vi "Spec Add.vi"(7 "프런트패널 윈도우:동작":T1(ring)=enum."Default", 8 "error in":errorcluster caption="에러 입력(에러 없음)", 11 "TBCALSPEC":string[][](table)) -> (0 "error out":errorcluster caption="에러 출력")   [LabVIEW 2020]
uses:
  Controls/Cmd_Spec Add.ctl
  Controls/Cmd_Mouse Popup.ctl
  Controls/Cmd_Read Query.ctl
  Controls/Clst_Query Info.ctl
  Controls/Cmd_Write Query.ctl
  <vilib>/Utility/miscctls.llb/LVRowAndColumnUnsignedTypeDef.ctl
  Variables/Global_Cal Info.vi
  Public/Polymorph/Array Dedup_1D Str.vi
  Public/Polymorph/Cell Space_Table.vi
  Public/Polymorph/Data Class_2D Str.vi
  <vilib>/addons/database/NI_Database_API.lvlib
panel:
  in  "번호정렬":bool
  in  "DB수정":bool
  in  "내용적용":bool
  in  "zero?":bool=TRUE caption="0점 10 digit 추가?"
  out "Data source":string[][](array[string])
  out "추가배열":string[](array[string])
  in  "새로 고침":bool
  in  "등록번호":string
  in  "빈칸\n줄임":bool
  in  "세부교정기능":string(combo)
  in  "교정기능":string(combo)
  in  "추가":bool
  in  "닫기":bool
  out "제조사명":string
  in  "제조사코드":string
  in  "모델":string
  out "기관명":string
  in  "DB등록":bool
  out "세부분류코드":string
  out "부서명":string
  in  "부서코드":string
  in  "기관코드":string
  in  "추가 단위":string(combo)
  in  "추가SPEC":string
  in  "Default 단위":string(combo)
  in  "Default 값":string
  out "슬라이드":i32(slide) scale=0.0..643.0
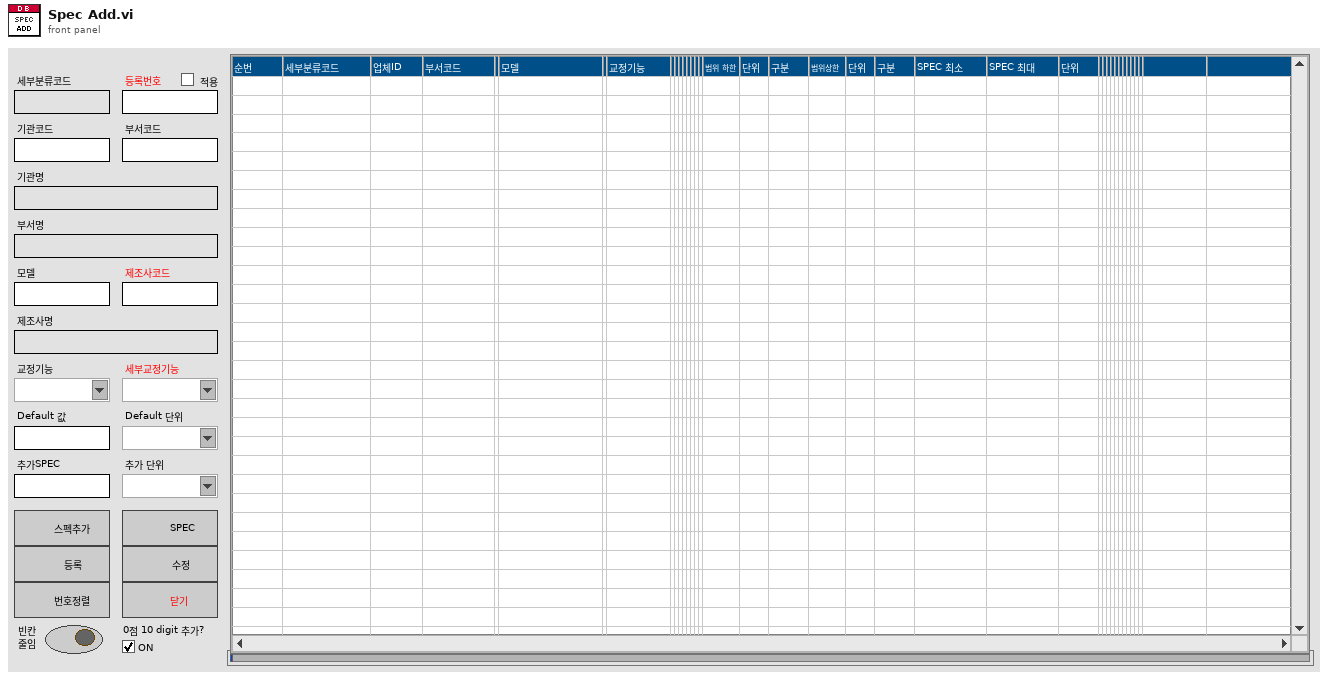
[diagram p1: front panel]
types:
  T1 = enum32{"Invalid", "Default", "Floating", "Floating/Auto-Hide", "Modal"}
  T2 = typedef "Cmd_Spec Add.ctl" = enum16{"Initialize", "Load Spec", "Wait Event", "Check data", "Create Row", "Add Spec", "Update Spec", "Error", "Exit"}
  T3 = typedef "Cmd_Mouse Popup.ctl" = enum16{"활성화", "메뉴선택"}
  T4 = cluster{"Shift":bool, "Ctrl":bool, "Alt":bool, "Cmd":bool, "Opt":bool}
  T5 = typedef "Clst_Query Info.ctl" = cluster{"사번":string, "등록번호":string, "업체명":string, "세부분류코드":string, "형식":string, "기기번호":string, "FUNC":string, "FUNC_EXT":string, "옵션":string, "추가문자열":string, "일자":string, "배열 1":string[], "배열 2":string[], "항목명":string, "문자열":string, "이름":string}
  T6 = typedef "Cmd_Read Query.ctl" = enum16{"교정자 이름 얻기", "인증교정자 얻기", "기술책임자 얻기", "기책부책 얻기", "등록번호 얻기", "등록정보 얻기", "업체정보 얻기", "교정일자(CAMAS) 얻기", "교정일자(CALSTD) 얻기", "교정환경 얻기", "교정절차서 목록 얻기", "교정절차서명 얻기", "교정절차 목록얻기", "교정절차 얻기", "PROC 교정절차 얻기", "PROC SPEC 얻기", "교정절차(Func별) 얻기", "교정절차(Func_ext별) 얻기", "기관코드 얻기", "교정기능(세부분류) 얻기", "교정기능(모델) 얻기", "교정기능 목록 얻기", "교정기능 명칭 얻기", "교정기능 항목명칭 얻기", "DB (사용기준기) 얻기", "DB (기준기이름) 얻기", "DB (기준기이름목록) 얻기", "DB (기준기목록) 얻기", "DB (기준기값) 얻기", "DB (CMC) 얻기", "DB (FUNC) 얻기", "DB (CALNAME) 얻기", "DB (STDNAME) 얻기", "DB (SPEC) 얻기", "모델(항목전체) 얻기", "모델(최대범위) 얻기", "모델(최소범위) 얻기", "모델(최대최소) 얻기", "모델(범위조건) 얻기", "모델(등록요청) 얻기", "모델(형식별) 얻기", "모델(조건별) 얻기", "모델(모델검색) 얻기", "세부분류 목록 얻기", "기준기등록리스트 얻기", "STD Cal Date Check", "DB등록일자 얻기", "적용항목 얻기", "기타정보 얻기", "기준기요청 얻기", "서버버전 얻기"}
  T7 = typedef "Cmd_Write Query.ctl" = enum16{"TBUSESTD_MCT Insert", "TBUSESTD_MCT Delete", "TBCALSTD_MCT_TEMP Insert", "TBCALSTD_MCT_TEMP Delete", "TBCALSTD_MCT Insert", "TBCALSTD_MCT Delete", "TBCALSTD_MCT_BACK Insert", "TBCALSTD_MCT_BACK Delete", "TBCALPROC_MCT Insert", "TBCALPROC_MCT Delete", "TBCALPROC_MCT_TEMP Insert", "TBCALPROC_MCT_TEMP Delete", "TBCALCMC_MCT Insert", "TBCALCMC_MCT Delete", "TBCALFUNC_MCT Insert", "TBCALFUNC_MCT Delete", "TBCALNAME_MCT Insert", "TBCALNAME_MCT Delete", "TBSTDNAME_MCT Insert", "TBSTDNAME_MCT Delete", "TBCALSPEC_MCT Insert", "TBCALSPEC_MCT Delete", "TBCALSTD_MCT NOTUSE update", "TBCALSPEC_MCT update", "TBMCTVERMAN update"}
  T8 = typedef "LVRowAndColumnUnsignedTypeDef.ctl" = cluster{"Row":u32, "Column":u32}
  T9 = typedef "Clst_Cal Info Global.ctl" = cluster{"등록번호":string, "의뢰기관":string, "기기명":string, "제작회사":string, "형식":string, "기기번호":string, "소분류코드":string, "세부분류코드":string, "교정주기":string, "접수번호":string, "교정일자":string, "교정절차서 1":string, "교정절차서 2":string, "교정절차서 3":string, "접수확인자":string, "인증교정자":string, "기술책임자":string, "KOLAS 유무":string, "진행상태":string, "의뢰기관코드":string, "입고형태":string, "영문성적서?":bool, "합불판정?":bool, "부록?":bool, "절차서번호 1":string, "절차서번호 2":string, "절차서번호 3":string, "교정방식":string, "부서명":string}
  T10 = typedef "NI_Database_API.lvlib/Conn ObjectReference.ctl" = refnum<k1>
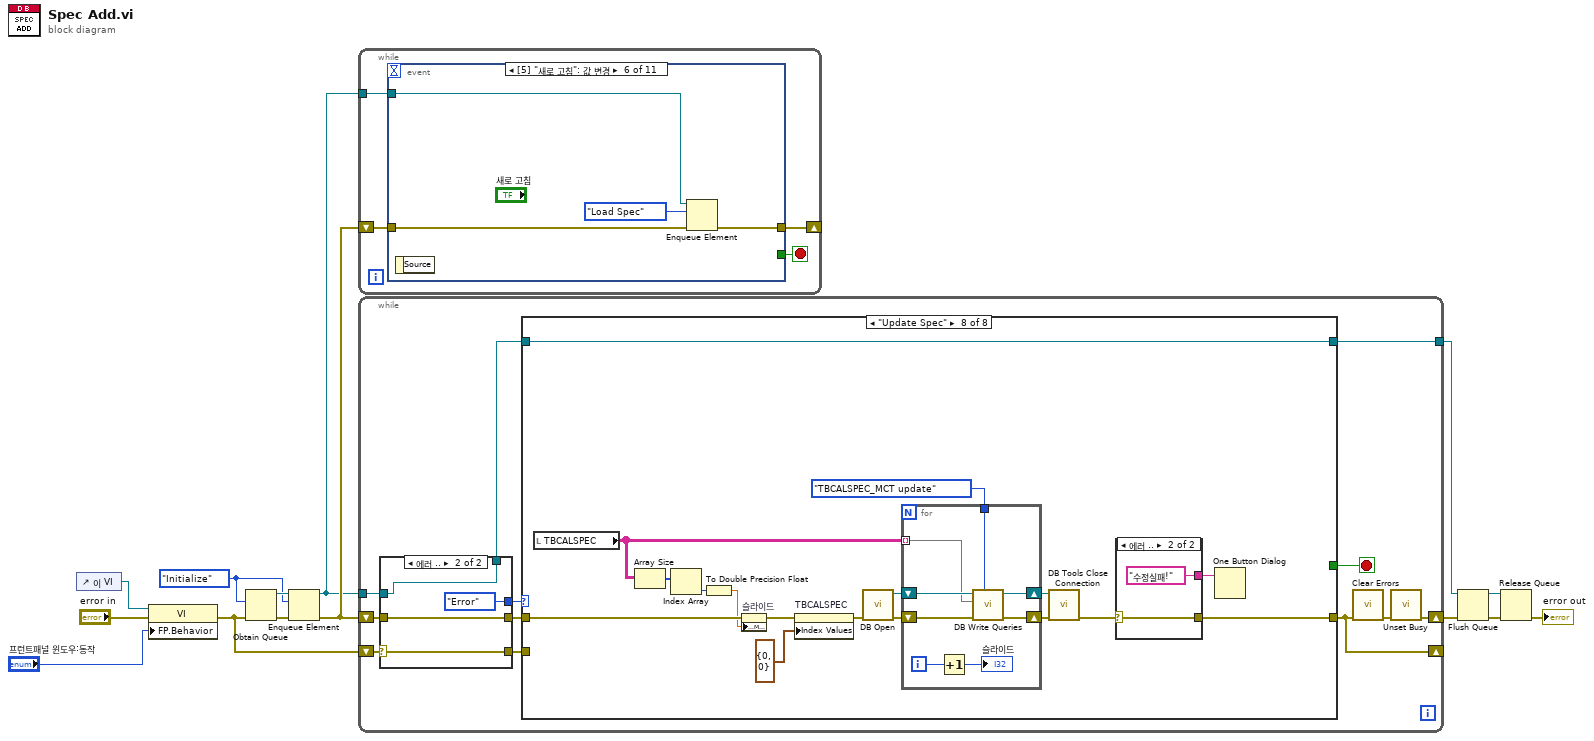
[diagram p0: block diagram]
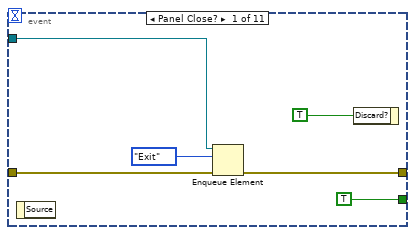
[diagram p2: hidden frame]
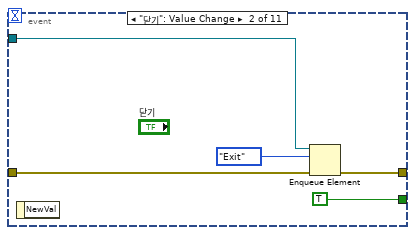
[diagram p3: hidden frame]
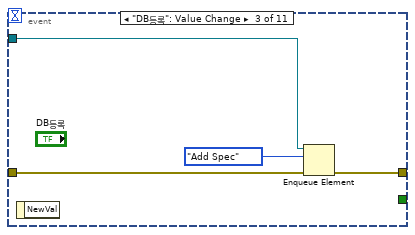
[diagram p4: hidden frame]
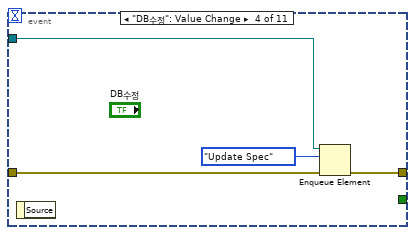
[diagram p5: hidden frame]
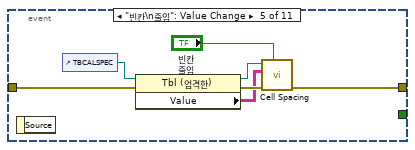
[diagram p6: hidden frame]
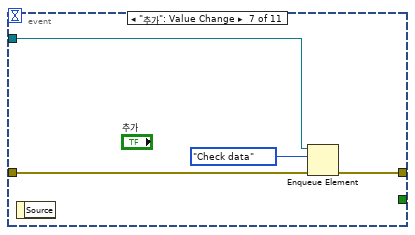
[diagram p7: hidden frame]
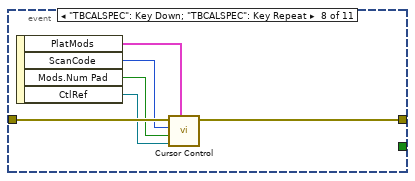
[diagram p8: hidden frame]
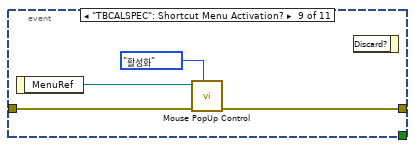
[diagram p9: hidden frame]
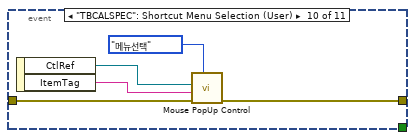
[diagram p10: hidden frame]
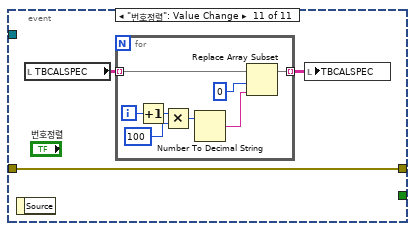
[diagram p11: hidden frame]
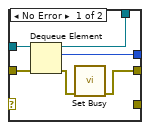
[diagram p12: hidden frame]
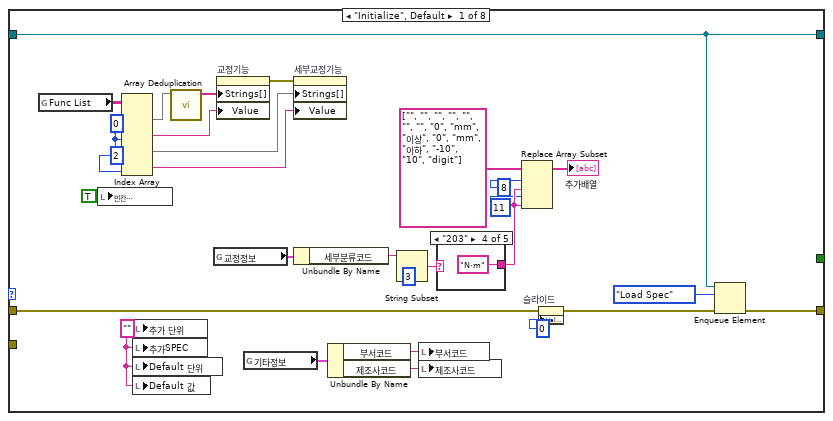
[diagram p13: hidden frame]
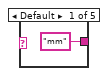
[diagram p14: hidden frame]
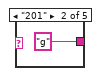
[diagram p15: hidden frame]
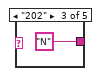
[diagram p16: hidden frame]
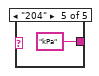
[diagram p17: hidden frame]
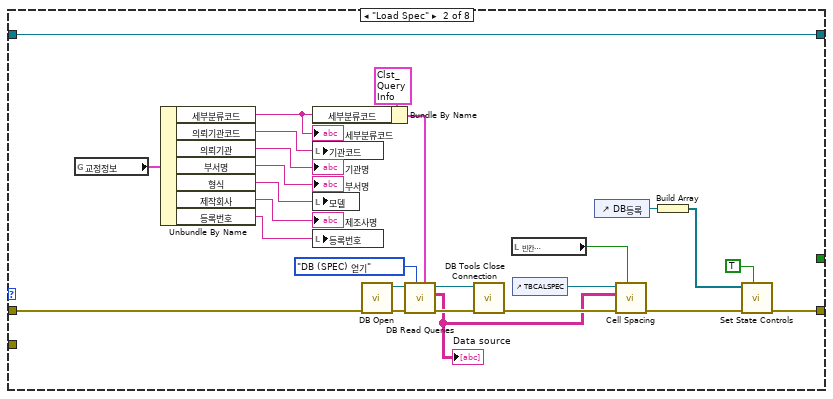
[diagram p18: hidden frame]
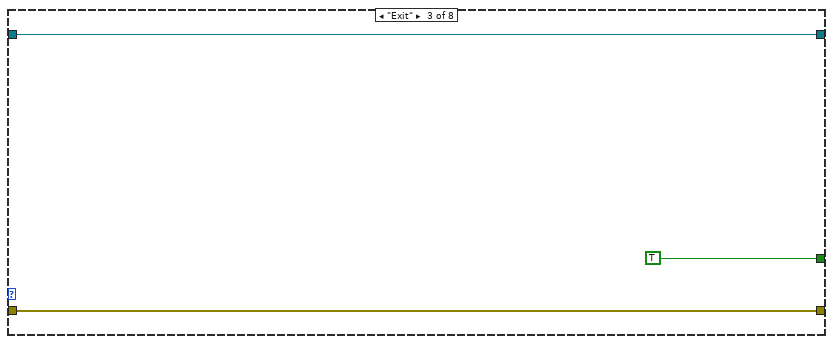
[diagram p19: hidden frame]
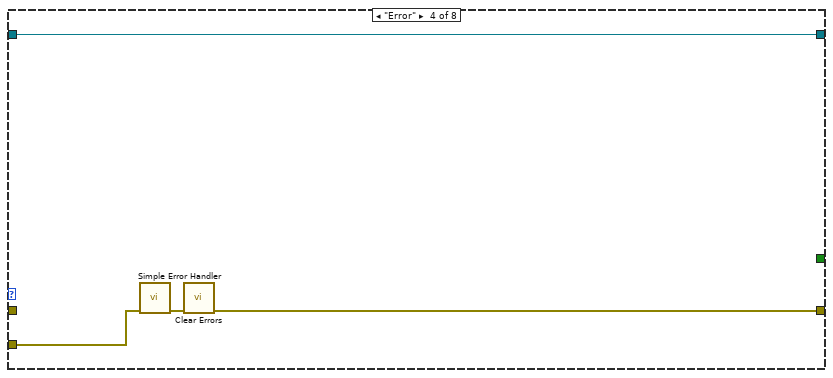
[diagram p20: hidden frame]
diagram:
  w6 = Cmd_Spec_Add."Initialize"
  n1 = control-ref of="이 VI"() -> (w2:refnum<vi>)
  n2 = property class="VI"(reference=w2, error in="error in", "FP.Behavior"="프런트패널 윈도우:동작") -> (error out=w3:errorcluster)  [unwired: 1 out]
  n3 = Obtain Queue(element data type=w6, error in (no error)=w3) -> (queue out=w10:refnum<queue>, error out=w9:errorcluster)  [unwired: 3 in, 1 out]
  n4 = Enqueue Element(queue=w10, element=w6, error in (no error)=w9) -> (queue out=w7:refnum<queue>, error out=w8:errorcluster)  [unwired: 1 in, 1 out]
  n5 = while {
    shift-right: [w16] -> _
    shift-left: w8 -> [w18]
    tunnel: w7 -> [w17]
    stop <- w15 stop-if-true
    n6 = event shown="[5] \"새로 고침\": 값 변경" {
      selector: _ -> [_ _ _ _ _ _ _ _ _ _ _]
      dyn-events: _ -> [_ _ _ _ _ _ _ _ _ _ _]
      timeout: _ -> [_ _ _ _ _ _ _ _ _ _ _]
      tunnel: w18 -> [w23 w29 w32 w36 w41 w47 w51 w57 w60 w65 w69]
      tunnel: [w22 w28 w32 w35 w43 w46 w50 w56 w59 w64 w69] -> w16
      tunnel: w17 -> [w21 w26 w31 w33 _ w45 w49 _ _ _ _]
      tunnel: [TRUE ("버림?") TRUE ("버림?") _ _ _ _ _ _ _ _ _] -> w15
      event Panel Close? {
        n7 = event-data() -> ()  [unwired: 1 in, 1 out]
        n8 = Enqueue Element(queue=w21, element=Cmd_Spec_Add."Exit", error in (no error)=w23) -> (error out=w22:errorcluster)  [unwired: 1 in, 2 out]
        n9 = event-data("Discard?"=TRUE ("버림?")) -> ()  [unwired: 1 in, 1 out]
      }
      event "닫기": Value Change {
        n10 = event-data() -> ()  [unwired: 1 in, 1 out]
        n11 = Enqueue Element(queue=w26, element=Cmd_Spec_Add."Exit", error in (no error)=w29) -> (error out=w28:errorcluster)  [unwired: 1 in, 2 out]
      }
      event "DB등록": Value Change {
        n12 = event-data() -> ()  [unwired: 1 in, 1 out]
        n13 = Enqueue Element(queue=w31, element=Cmd_Spec_Add."Add Spec", error in (no error)=w32) -> ()  [unwired: 1 in, 3 out]
      }
      event "DB수정": Value Change {
        n14 = event-data() -> ()  [unwired: 1 in, 1 out]
        n15 = Enqueue Element(queue=w33, element=Cmd_Spec_Add."Update Spec", error in (no error)=w36) -> (error out=w35:errorcluster)  [unwired: 1 in, 2 out]
      }
      event "빈칸\n줄임": Value Change {
        n16 = event-data() -> ()  [unwired: 1 in, 1 out]
        n17 = control-ref of="TBCALSPEC"() -> (w38:refnum<vi>)
        n18 = property class="Tbl (엄격한)"(reference=w38, error in=w41) -> (reference out=w37:refnum<vi>, error out=w40:errorcluster, "Value"=w39:string[][])
        n19 = call-poly "Cell Spacing.vi"("빈내용 숨기기?(F)"="빈칸\n줄임", "error in"=w40, "Data in"=w39, "테이블 참조 in"=w37) -> ("error out"=w43:errorcluster)  [unwired: 5 in, 2 out]
      }
      event "새로 고침": Value Change {
        n20 = event-data() -> ()  [unwired: 1 in, 1 out]
        n21 = Enqueue Element(queue=w45, element=Cmd_Spec_Add."Load Spec", error in (no error)=w47) -> (error out=w46:errorcluster)  [unwired: 1 in, 2 out]
      }
      event "추가": Value Change {
        n22 = event-data() -> ()  [unwired: 1 in, 1 out]
        n23 = Enqueue Element(queue=w49, element=Cmd_Spec_Add."Check data", error in (no error)=w51) -> (error out=w50:errorcluster)  [unwired: 1 in, 2 out]
      }
      event "TBCALSPEC": Key Down; "TBCALSPEC": Key Repeat {
        n24 = event-data() -> ("PlatMods"=w55:T4, "ScanCode"=w54:i16, "Mods.Num Pad"=w53:bool, "CtlRef"=w52:refnum<vi>)  [unwired: 1 in]
        n25 = call "Cursor Control.vi"("플랫폼 조합키"=w55, "참조"=w52, "Num Pad"=w53, "ScanCode"=w54, "error in"=w57) -> ("error out"=w56:errorcluster)  [unwired: 5 in, 1 out]
      }
      event "TBCALSPEC": Shortcut Menu Activation? {
        n26 = event-data() -> ("MenuRef"=w58:refnum<k9>)  [unwired: 1 in]
        n27 = call "Mouse PopUp Control.vi"("type"=Cmd_Mouse_Popup."활성화", "error in"=w60, "메뉴 참조"=w58) -> ("error out"=w59:errorcluster)  [unwired: 8 in]
        n28 = event-data() -> ()  [unwired: 2 in, 1 out]
      }
      event "TBCALSPEC": Shortcut Menu Selection (User) {
        n29 = event-data() -> ("CtlRef"=w63:refnum<vi>, "ItemTag"=w62:string)  [unwired: 1 in]
        n30 = call "Mouse PopUp Control.vi"("type"=Cmd_Mouse_Popup."메뉴선택", "error in"=w65, "아이템 태그"=w62, "Tbl 참조 번호"=w63) -> ("error out"=w64:errorcluster)  [unwired: 7 in]
      }
      event "번호정렬": Value Change {
        n31 = event-data() -> ()  [unwired: 1 in, 1 out]
        n32 = local read "TBCALSPEC"() -> (w68:string[][])
        n33 = for {
          tunnel: w68 -> [w73] mode=indexing
          tunnel: [w70] -> w67 mode=indexing
          i -> [w77]
          n34 = Increment(x=w77) -> (x+1=w76:i32)
          n35 = Multiply(x=w76, y=100) -> (x*y=w74:i32)
          n36 = Number To Decimal String(number=w74) -> (decimal integer string=w71:string)  [unwired: 1 in]
          n37 = Replace Array Subset(array=w73, new element=w71, index=0 ("인덱스")) -> (w70:string[])
        }
        n38 = local write "TBCALSPEC"(w67) -> ()
      }
    }
  }
  n39 = while {
    shift-right: [w82] -> w14
    shift-left: w8 -> [w89]
    tunnel: w7 -> [w88]
    shift-right: [w81] -> _
    shift-left: w3 -> [w80]
    tunnel: [w78] -> w5
    stop <- w86 stop-if-true
    n40 = case shown="에러 .." w80 {
      selector: w80 -> [_ w97]
      tunnel: w89 -> [w95 w99]
      tunnel: w88 -> [w94 w96]
      tunnel: [w93 Cmd_Spec_Add."Error"] -> w87
      tunnel: [w91 w99] -> w85
      tunnel: [w90 w96] -> w83
      tunnel: [_ w97] -> w79
      frame No Error {
        n41 = Dequeue Element(queue=w94, error in (no error)=w95) -> (queue out=w90:refnum<queue>, element=w93:T2, error out=w92:errorcluster)  [unwired: 1 in, 1 out]
        n42 = call <vilib>:"Set Busy.vi"("error in (no error)"=w92) -> ("error out"=w91:errorcluster)  [unwired: 9 in, 1 out]
      }
      frame Error {
      }
    }
    n43 = case shown="\"Update Spec\"" w87 {
      tunnel: [_ _ TRUE ("취소") _ _ _ _ _] -> w86
      tunnel: w85 -> [w102 w143 w162 _ w169 w219 w259 w340]
      tunnel: [w105 w134 w162 w165 w177 w218 w261 w343] -> w81
      tunnel: w83 -> [w103 w140 w160 w163 w176 w217 w269 w341]
      tunnel: w79 -> [_ _ _ w164 _ _ _ _]
      tunnel: [w103 w140 w160 w163 w176 w217 w269 w341] -> w78
      frame "Initialize", Default {
        w118 = "" ("추가 단위")
        w121 = 2 ("인덱스 (열)")
        w120 = 0 ("비활성화된 인덱스 (열)")
        n44 = global read "Global_Cal Info.vi" "Func List"() -> (w127:string[][])
        n45 = local write "빈칸\n줄임"(TRUE ("빈내용 숨기기?(F)")) -> ()
        n46 = Index Array(array=w127, index (col) #1=w120, index (row) #2=w120, index (col) #2=w120, index (col) #3=w121, index (row) #4=w120, index (col) #4=w121) -> (element #1=w125:string[], element #2=w126:string, element #3=w122:string[], element #4=w119:string)  [unwired: 2 in]
        n47 = local write "추가 단위"(w118) -> ()
        n48 = local write "추가SPEC"(w118) -> ()
        n49 = local write "Default 단위"(w118) -> ()
        n50 = local write "Default 값"(w118) -> ()
        n51 = call-poly "Array Deduplication.vi"("배열 in"=w125) -> ("배열 out"=w124:string[])  [unwired: 9 in, 1 out]
        n52 = global read "Global_Cal Info.vi" "교정정보"() -> (w111:T9)
        n53 = property on="교정기능" class="CmbBox"("Strings[]"=w124, "Value"=w126) -> (error out=w123:errorcluster)  [unwired: 2 in, 1 out]
        n54 = global read "Global_Cal Info.vi" "기타정보"() -> (w128:cluster{"부서코드":string, "제조사코드":string})
        n55 = property on="세부교정기능" class="CmbBox"(error in=w123, "Strings[]"=w122, "Value"=w119) -> ()  [unwired: 1 in, 2 out]
        n56 = Unbundle By Name(w111) -> ("세부분류코드"=w112:string)
        n57 = Unbundle By Name(w128) -> ("부서코드"=w117:string, "제조사코드"=w116:string)
        n58 = String Subset(string=w112, length (rest)=3 ("길이(나머지)")) -> (substring=w113:string)  [unwired: 1 in]
        n59 = local write "부서코드"(w117) -> ()
        n60 = local write "제조사코드"(w116) -> ()
        n61 = case shown="\"203\"" w113 {
          tunnel: ["mm" "g" "N" "N·m" "kPa"] -> w114
          frame Default {
          }
          frame "201" {
          }
          frame "202" {
          }
          frame "203" {
          }
          frame "204" {
          }
        }
        n62 = Replace Array Subset(array=string[] ["", "", "", "", "", "", "", "0", "mm", "이상", "0", "mm", "이하", "-10", "10", "digit"], new element #1=w114, index #1=8 ("인덱스"), new element #2=w114, index #2=11 ("인덱스")) -> (→"추가배열":string[])
        n63 = property on="슬라이드" class="Slide (엄격한)"(error in=w102, "Value"=0 ("슬라이드")) -> (error out=w101:errorcluster)  [unwired: 1 in, 1 out]
        n64 = Enqueue Element(queue=w103, element=Cmd_Spec_Add."Load Spec", error in (no error)=w101) -> (error out=w105:errorcluster)  [unwired: 1 in, 2 out]
      }
      frame "Load Spec" {
        n65 = global read "Global_Cal Info.vi" "교정정보"() -> (w156:T9)
        n66 = Unbundle By Name(w156) -> ("세부분류코드"=w154:string, "의뢰기관코드"=w147:string, "의뢰기관"=→"기관명":string, "부서명"=→"부서명":string, "형식"=w141:string, "제작회사"=→"제조사명":string, "등록번호"=w146:string)
        "세부분류코드" <- w154
        n67 = Bundle By Name(cluster=T5 {"사번"="", "등록번호"="", "업체명"="", "세부분류코드"="", "형식"="", "기기번호"="", "FUNC"="", "FUNC_EXT"="", "옵션"="", "추가문자열"="", "일자"="", "배열 1"=[], "배열 2"=[], "항목명"="", "문자열"="", "이름"=""} ("Query info"), "세부분류코드"=w154) -> (w155:T5)
        n68 = local write "기관코드"(w147) -> ()
        n69 = local write "모델"(w141) -> ()
        n70 = local write "등록번호"(w146) -> ()
        n71 = call "DB Open.vi"("에러 입력"=w143) -> ("에러 출력"=w142:errorcluster, "참조 번호 출력"=w159:T10)  [unwired: 9 in]
        n72 = call "DB Read Queries.vi"("Query info"=w155, "Query Command"=Cmd_Read_Query."DB (SPEC) 얻기", "에러 입력(에러 없음)"=w142, "참조 번호 입력"=w159) -> ("에러 출력"=w157:errorcluster, "Data"=w139:string[][], "참조 번호 출력"=w158:T10)  [unwired: 3 in, 2 out]
        "Data source" <- w139
        n73 = call <vilib>:"DB Tools Close Connection.vi"("error in (no error)"=w157, "connection reference"=w158) -> ("error out"=w149:errorcluster)  [unwired: 5 in]
        n74 = local read "빈칸\n줄임"() -> (w148:bool)
        n75 = control-ref of="TBCALSPEC"() -> (w150:refnum<vi>)
        n76 = control-ref of="DB등록"() -> (w138:refnum<vi>)
        n77 = call-poly "Cell Spacing.vi"("빈내용 숨기기?(F)"=w148, "error in"=w149, "Data in"=w139, "테이블 참조 in"=w150) -> ("error out"=w135:errorcluster)  [unwired: 5 in, 2 out]
        n78 = Build Array(w138) -> (w137:refnum<vi>[])
        n79 = call "Set State Controls.vi"("활성화 (F)"=TRUE, "error in (no error)"=w135, "컨트롤 참조 배열 in"=w137) -> ("error out"=w134:errorcluster)  [unwired: 7 in, 1 out]
      }
      frame "Exit" {
      }
      frame "Error" {
        n80 = call <vilib>:"Simple Error Handler.vi"("error in (no error)"=w164) -> ("error out"=w166:errorcluster)  [unwired: 4 in, 4 out]
        n81 = call <vilib>:"Clear Errors.vi"("error in (no error)"=w166) -> ("error out"=w165:errorcluster)  [unwired: 5 in, 1 out]
      }
      frame "Add Spec" {
        n82 = local read "Data source"() -> (w175:string[][])
        n83 = local read "TBCALSPEC"() -> (w170:string[][])
        n84 = Array Size(array=w170) -> (size(s)=w168:i32[])
        n85 = Concatenate Strings(w175) -> (w174:string)
        n86 = Concatenate Strings(w170) -> (w173:string)
        n87 = Equal?(x=w174, y=w173) -> (x = y?=w172:bool)
        n88 = Index Array(array=w168) -> (element=w167:i32)  [unwired: 1 in]
        n89 = case shown="거짓" w172 {
          tunnel: w169 -> [w181 w212]
          tunnel: [w193 w212] -> w177
          tunnel: w170 -> [w183 _]
          tunnel: [w182 "DB 내용과 같습니다."] -> w171
          tunnel: w167 -> [w179 _]
          frame False {
            n90 = To Double Precision Float(number=w179) -> (double precision float=w178:dbl)
            n91 = local read "세부분류코드"() -> (w184:string)
            n92 = property on="슬라이드" class="Slide (엄격한)"(error in=w181, "Scale.Maximum"=w178) -> (error out=w180:errorcluster)  [unwired: 1 in, 1 out]
            n93 = property on="TBCALSPEC" class="Tbl (엄격한)"(error in=w180, "Index Values"=T8 {"Row"=0, "Column"=0} ("인덱스 값")) -> (error out=w187:errorcluster)  [unwired: 1 in, 1 out]
            n94 = Bundle By Name(cluster=T5 {"사번"="", "등록번호"="", "업체명"="", "세부분류코드"="", "형식"="", "기기번호"="", "FUNC"="", "FUNC_EXT"="", "옵션"="", "추가문자열"="", "일자"="", "배열 1"=[], "배열 2"=[], "항목명"="", "문자열"="", "이름"=""} ("Query info"), "세부분류코드"=w184) -> (w185:T5)
            n95 = call "DB Open.vi"("에러 입력"=w187) -> ("에러 출력"=w191:errorcluster, "참조 번호 출력"=w192:T10)  [unwired: 9 in]
            n96 = call "DB Write Queries.vi"("Query info"=w185, "COMMAND"=Cmd_Write_Query."TBCALSPEC_MCT Delete", "에러 입력(에러 없음)"=w191, "참조 번호 입력"=w192) -> ("에러 출력"=w189:errorcluster, "참조 번호 출력"=w190:T10)  [unwired: 6 in]
            n97 = for {
              tunnel: Cmd_Write_Query."TBCALSPEC_MCT Insert" ("COMMAND") -> [w210]
              tunnel: w183 -> [w203] mode=indexing
              shift-right: [w207] -> w196
              shift-left: w189 -> [w209]
              shift-right: [w206] -> w195
              shift-left: w190 -> [w208]
              i -> [w205]
              n98 = Increment(x=w205) -> (x+1=w204:i32)
              n99 = call "DB Write Queries.vi"("COMMAND"=w210, "에러 입력(에러 없음)"=w209, "DATA IN"=w203, "참조 번호 입력"=w208) -> ("에러 출력"=w207:errorcluster, "참조 번호 출력"=w206:T10)  [unwired: 6 in]
              n100 = property on="슬라이드" class="Slide (엄격한)"("Value"=w204) -> ()  [unwired: 2 in, 2 out]
            }
            n101 = call <vilib>:"DB Tools Close Connection.vi"("error in (no error)"=w196, "connection reference"=w195) -> ("error out"=w194:errorcluster)  [unwired: 5 in]
            n102 = case shown="에러 없음" w194 {
              selector: w194 -> [w199 w201]
              tunnel: [w199 w201] -> w193
              tunnel: ["등록성공!" "등록실패!"] -> w182
              frame No Error {
              }
              frame Error {
              }
            }
          }
          frame True {
          }
        }
        n103 = One Button Dialog(message=w171) -> ()  [unwired: 1 in, 1 out]
      }
      frame "Check data" {
        n104 = local read "내용적용"() -> (w213:bool)
        n105 = case shown="참" w213 {
          tunnel: [_ w230] -> w216
          tunnel: [_ w229] -> w215
          tunnel: [_ w228] -> w214
          frame False {
          }
          frame True {
            n106 = local read "세부교정기능"() -> (w228:string)
            n107 = local read "제조사코드"() -> (w229:string)
            n108 = local read "등록번호"() -> (w230:string)
          }
        }
        n109 = local read "기관코드"() -> (w224:string)
        n110 = local read "부서코드"() -> (w225:string)
        n111 = local read "교정기능"() -> (w227:string)
        n112 = local read "TBCALSPEC"() -> (w222:string[][])
        n113 = local read "모델"() -> (w226:string)
        n114 = Build Array(w224, w225, w216, w226, w215, w227, w214) -> (w223:string[])
        n115 = for {
          tunnel: w223 -> [w247] mode=indexing
          shift-right: [w248] -> w220
          shift-left: w222 -> [w249]
          i -> [w250]
          n116 = case shown="기본" w247 {
            selector: w247 -> [_ w252]
            tunnel: w250 -> [_ w257]
            tunnel: w249 -> [w251 w256]
            tunnel: [w251 w255] -> w248
            frame "" {
            }
            frame Default {
              n117 = Add(x=w257, y=2) -> (x+y=w254:i32)
              n118 = call-poly "Data Classification.vi"("인덱스"=w254, "DATA 입력"=w256, "검색 문자열"=w252) -> ("DATA 출력"=w255:string[][])  [unwired: 4 in, 4 out]
            }
          }
        }
        n119 = Empty Array?(array=w220) -> (empty?=w221:bool)
        n120 = case shown="거짓" w221 {
          tunnel: w220 -> [w240 _]
          tunnel: w219 -> [w241 w246]
          tunnel: [w233 w243] -> w218
          tunnel: w217 -> [_ w245]
          frame False {
            n121 = control-ref of="DB수정"() -> (w238:refnum<vi>)
            n122 = property on="TBCALSPEC" class="Tbl (엄격한)"(error in=w241, "Value"=w240, "Index Values"=T8 {"Row"=0, "Column"=0} ("인덱스 값")) -> (error out=w235:errorcluster)  [unwired: 1 in, 1 out]
            n123 = control-ref of="DB등록"() -> (w232:refnum<vi>)
            n124 = Build Array(w238) -> (w237:refnum<vi>[])
            n125 = One Button Dialog(message="해당 spec 존재!" ("메시지")) -> ()  [unwired: 1 in, 1 out]
            n126 = call "Set State Controls.vi"("활성화 (F)"=TRUE, "error in (no error)"=w235, "컨트롤 참조 배열 in"=w237) -> ("error out"=w234:errorcluster)  [unwired: 7 in, 1 out]
            n127 = Build Array(w232) -> (w231:refnum<vi>[])
            n128 = call "Set State Controls.vi"("error in (no error)"=w234, "컨트롤 참조 배열 in"=w231) -> ("error out"=w233:errorcluster)  [unwired: 8 in, 1 out]
          }
          frame True {
            n129 = Enqueue Element(queue=w245, element=Cmd_Spec_Add."Create Row", error in (no error)=w246) -> (error out=w243:errorcluster)  [unwired: 1 in, 2 out]
          }
        }
      }
      frame "Create Row" {
        n130 = Index Array(array="TBCALSPEC", index (col)=0 ("비활성화된 인덱스 (열)")) -> (element=w305:string[])  [unwired: 1 in]
        n131 = case shown="참" "내용적용" {
          tunnel: [_ "제조사코드"] -> w297
          tunnel: [_ "등록번호"] -> w296
          tunnel: [_ "세부교정기능"] -> w294
          frame False {
          }
          frame True {
          }
        }
        n132 = Reverse 1D Array(array=w305) -> (reversed array=w304:string[])
        n133 = Index Array(array=w304) -> (element=w303:string)  [unwired: 1 in]
        n134 = Decimal String To Number(string=w303) -> (number=w276:i32)  [unwired: 2 in, 1 out]
        n135 = local read "세부분류코드"() -> (w300:string)
        n136 = Add(x=w276, y=100) -> (x+y=w302:i32)
        n137 = Number To Decimal String(number=w302) -> (decimal integer string=w273:string)  [unwired: 1 in]
        n138 = Add(x=w276, y=200) -> (x+y=w274:i32)
        n139 = Concatenate Strings("-" ("문자열"), "Default 값") -> (w285:string)
        n140 = Number To Decimal String(number=w274) -> (decimal integer string=w272:string)  [unwired: 1 in]
        n141 = Build Array(w300, "기관코드", "부서코드", w296, "모델", w297, "교정기능", w294) -> (w278:string[])
        n142 = Build Array(w285, "Default 값", "Default 단위", "추가SPEC", "추가 단위") -> (w281:string[])
        n143 = Build Array (concatenate)(w278, string[] ["", "", "", "", "", "", "", "", "", "", "", "", ""], w281) -> (w271:string[])
        n144 = Array Size(array="TBCALSPEC") -> (size(s)=w301:i32[])
        n145 = case shown="참" "zero?" {
          tunnel: "TBCALSPEC" -> [w315 w334]
          tunnel: [w314 w333] -> w263
          tunnel: w278 -> [w313 _]
          tunnel: "Default 단위" -> [w312 _]
          tunnel: w273 -> [w311 w332]
          tunnel: w272 -> [w310 _]
          tunnel: w271 -> [w309 w331]
          frame True {
            n146 = case shown="\"%\"" w312 {
              tunnel: w315 -> [w320 w329]
              tunnel: [w319 w328] -> w314
              tunnel: w313 -> [_ w327]
              tunnel: w311 -> [w316 w325]
              tunnel: w310 -> [_ w324]
              tunnel: w309 -> [w317 w323]
              frame Default {
                n147 = Build Array (concatenate)(w316, w317) -> (w318:string[])
                n148 = Insert Into Array(array=w320, new element=w318) -> (w319:string[][])  [unwired: 2 in]
              }
              frame "%" {
                n149 = local read "추가배열"() -> (w321:string[])
                n150 = Build Array (concatenate)(w324, w323) -> (w322:string[])
                n151 = Build Array (concatenate)(w325, w327, w321) -> (w326:string[])
                n152 = Insert Into Array(array=w329, new element #1=w326, new element #2=w322) -> (w328:string[][])  [unwired: 2 in]
              }
            }
          }
          frame False {
            n153 = Build Array (concatenate)(w332, w331) -> (w330:string[])
            n154 = Insert Into Array(array=w334, new element=w330) -> (w333:string[][])  [unwired: 2 in]
          }
        }
        n155 = Index Array(array=w301) -> (element=w283:i32)  [unwired: 1 in]
        n156 = Subtract(x=w283, y=5) -> (x-y=w268:i32)
        n157 = Max & Min(x=0, y=w268) -> (max(x,y)=w267:i32)  [unwired: 1 out]
        n158 = Bundle(w267, 0) -> (w282:cluster{i32, i32})  [unwired: 1 in]
        n159 = local read "빈칸\n줄임"() -> (w264:bool)
        n160 = control-ref of="TBCALSPEC"() -> (w265:refnum<vi>)
        n161 = call-poly "Cell Spacing.vi"("빈내용 숨기기?(F)"=w264, "error in"=w259, "Data in"=w263, "테이블 참조 in"=w265) -> ("error out"=w262:errorcluster, "테이블 참조 Out"=w260:refnum<vi>)  [unwired: 5 in, 1 out]
        n162 = property on="프로퍼티 노드" class="Tbl"(reference=w260, error in=w262, "Index Values"=w282) -> (error out=w261:errorcluster)  [unwired: 1 out]
      }
      frame "Update Spec" {
        n163 = local read "TBCALSPEC"() -> (w338:string[][])
        n164 = Array Size(array=w338) -> (size(s)=w337:i32[])
        n165 = Index Array(array=w337) -> (element=w336:i32)  [unwired: 1 in]
        n166 = To Double Precision Float(number=w336) -> (double precision float=w335:dbl)
        n167 = property on="슬라이드" class="Slide (엄격한)"(error in=w340, "Scale.Maximum"=w335) -> (error out=w339:errorcluster)  [unwired: 1 in, 1 out]
        n168 = property on="TBCALSPEC" class="Tbl (엄격한)"(error in=w339, "Index Values"=T8 {"Row"=0, "Column"=0} ("인덱스 값")) -> (error out=w350:errorcluster)  [unwired: 1 in, 1 out]
        n169 = call "DB Open.vi"("에러 입력"=w350) -> ("에러 출력"=w348:errorcluster, "참조 번호 출력"=w347:T10)  [unwired: 9 in]
        n170 = for {
          tunnel: Cmd_Write_Query."TBCALSPEC_MCT update" ("COMMAND") -> [w363]
          tunnel: w338 -> [w358] mode=indexing
          shift-right: [w360] -> w346
          shift-left: w348 -> [w362]
          shift-right: [w359] -> w345
          shift-left: w347 -> [w361]
          i -> [w357]
          n171 = Increment(x=w357) -> (x+1=→"슬라이드":i32)
          n172 = call "DB Write Queries.vi"("COMMAND"=w363, "에러 입력(에러 없음)"=w362, "DATA IN"=w358, "참조 번호 입력"=w361) -> ("에러 출력"=w360:errorcluster, "참조 번호 출력"=w359:T10)  [unwired: 6 in]
        }
        n173 = call <vilib>:"DB Tools Close Connection.vi"("error in (no error)"=w346, "connection reference"=w345) -> ("error out"=w344:errorcluster)  [unwired: 5 in]
        n174 = case shown="에러 .." w344 {
          selector: w344 -> [w353 w354]
          tunnel: [w353 w354] -> w343
          tunnel: ["수정성공!" "수정실패!"] -> w342
          frame No Error {
          }
          frame Error {
          }
        }
        n175 = One Button Dialog(message=w342) -> ()  [unwired: 1 in, 1 out]
      }
    }
    n176 = call <vilib>:"Clear Errors.vi"("error in (no error)"=w81) -> ("error out"=w84:errorcluster)  [unwired: 5 in, 1 out]
    n177 = call <vilib>:"Unset Busy.vi"("error in (no error)"=w84) -> ("error out"=w82:errorcluster)  [unwired: 10 in]
  }
  n178 = Flush Queue(queue=w5, error in (no error)=w14) -> (queue out=w12:refnum<queue>, error out=w13:errorcluster)  [unwired: 1 out]
  n179 = Release Queue(queue=w12, error in (no error)=w13) -> (error out=→"error out":errorcluster)  [unwired: 1 in, 2 out]
